vi "Set Resolution.vi"(8 "error in":errorcluster, 11 "IMG_SRC in":refnum<class "IMG_SRC.lvclass">) -> (0 "error out":errorcluster, 2 "Supported?":bool, 3 "IMG_SRC out":refnum<class "IMG_SRC.lvclass">)   [LabVIEW 2018, in "IMG_SRC.lvlib" / "IMG_SRC.lvclass"]
uses:
  IMG_SRC.lvclass
  IMG_SRC.lvclass/IMG_SRC.ctl
  builds/Camera.lvlibp/Camera.lvclass
  C:/Users/Ron.Dexter.LUMINARTECH/Desktop/builds/Camera.lvlibp/Camera.lvclass
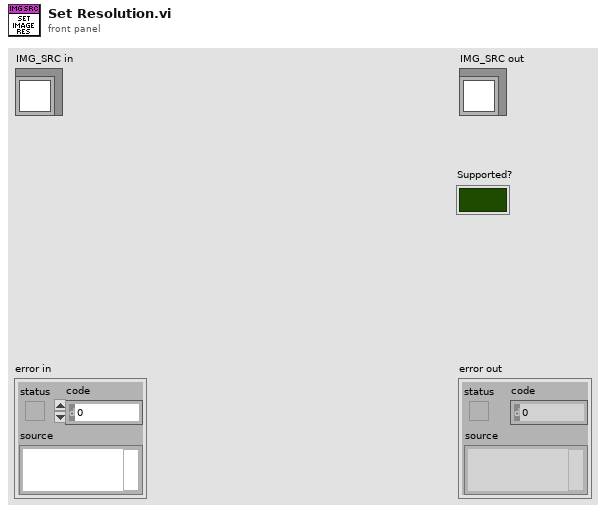
[diagram p1: front panel]
types:
  T1 = typedef "Camera.lvlibp/Camera.lvclass/Image Resolution.ctl" = enum16{"640x480", "1024x768", "1280x720", "1280x1024", "1600x1200", "1920x1080", "1920x1200"}
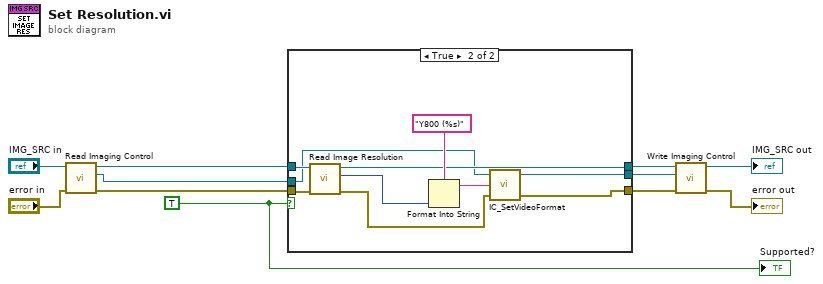
[diagram p0: block diagram]
diagram:
  w1 = TRUE
  n1 = call "Read Imaging Control.vi"("error in (no error)"="error in", "IMG_SRC in"="IMG_SRC in") -> ("error out"=w2:errorcluster, "Imaging Control"=w3:refnum<k7>, "IMG_SRC out"=w9:refnum<class "IMG_SRC.lvclass">)  [unwired: 7 in]
  n2 = case shown="True" w1 {
    tunnel: w9 -> [w12 w20]
    tunnel: w3 -> [w13 w15]
    tunnel: w2 -> [w14 w19]
    tunnel: [w12 w17] -> w6
    tunnel: [w13 w18] -> w5
    tunnel: [w14 w16] -> w4
    frame False {
    }
    frame True {
      n3 = call "Read Image Resolution.vi"("error in (no error)"=w19, "Camera in"=w20) -> ("error out"=w24:errorcluster, "Image Resolution"=w21:T1, "Camera out"=w17:refnum<class "IMG_SRC.lvclass">)  [unwired: 7 in]
      n4 = Format Into String(format string="Y800 (%s)", w21) -> (resulting string=w23:string)  [unwired: 2 in, 1 out]
      n5 = call <userlib>:"IC_SetVideoFormat.vi"("Error In (no error)"=w24, "VideoFormat"=w23, "ICImagingControl In"=w15) -> ("Error Out"=w16:errorcluster, "ICImagingControl Out"=w18:refnum<k7>)  [unwired: 1 out]
    }
  }
  n6 = call "Write Imaging Control.vi"("error in (no error)"=w4, "Imaging Control"=w5, "IMG_SRC in"=w6) -> ("error out"=→"error out":errorcluster, "IMG_SRC out"=→"IMG_SRC out":refnum<class "IMG_SRC.lvclass">)  [unwired: 7 in]
  "Supported?" <- w1
